vi "TESynC Example.vi"() -> ()   [LabVIEW 2010]
panel:
  in  "VISA resource name":refnum<visa-resource-name>
  out "Alarms":string
  out "Event State Readback(1=ON,0=OFF)":bool
  in  "Event State":bool
  in  "Event number":u8
  out "Actual Humidity Readback (%)":dbl format="%.2f"
  out "Setpoint Humidity Readback(%)":dbl format="%.2f"
  in  "Humidity Setpoint(%)":dbl format="%.2f"
  out "Actual Temp Readback (C)":dbl format="%.2f"
  out "Chamber State Readback(1=ON,0=OFF) 2":bool
  out "Chamber (1=ON,0=OFF)":bool
  in  "Temperature (C":dbl format="%.2f"
  out "Temp Setpoint Readback(C)":dbl format="%.2f"
  out "error out":errorcluster {"code" format="%.0x"}
  in  "error in (no error)":errorcluster
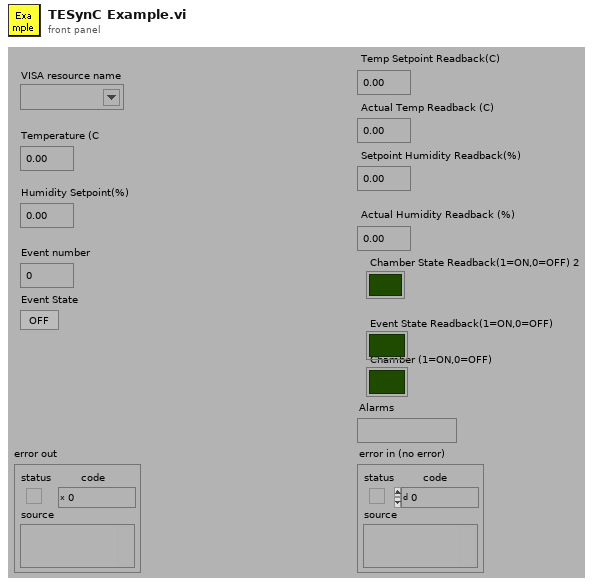
[diagram p1: front panel]
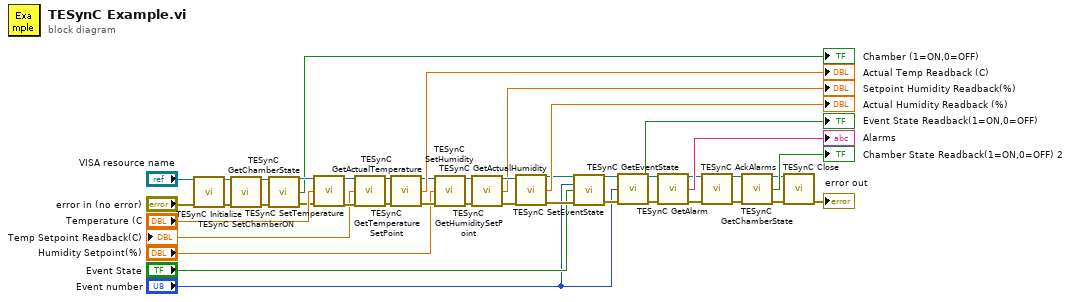
[diagram p0: block diagram]
diagram:
  n1 = call "TESynC Initialize.vi"("VISA resource name"="VISA resource name", "error in (no error)"="error in (no error)") -> ("VISA session"=w37:refnum<visa-resource-name>, "error out"=w38:errorcluster)  [unwired: 12 in]
  n2 = call "TESynC SetChamberON.vi"("VISA session in"=w37, "error in (no error)"=w38) -> ("VISA session out"=w35:refnum<visa-resource-name>, "error out"=w36:errorcluster)  [unwired: 12 in]
  n3 = call "TESynC GetChamberState.vi"("VISA session in"=w35, "error in (no error)"=w36) -> ("VISA session out"=w34:refnum<visa-resource-name>, "Chamber State Readback (1=ON,0=OFF)"=→"Chamber (1=ON,0=OFF)":bool, "error out"=w33:errorcluster)  [unwired: 11 in]
  n4 = call "TESynC SetTemperature.vi"("VISA session in"=w34, "Temperature (C"="Temperature (C", "error in (no error)"=w33) -> ("VISA session out"=w41:refnum<visa-resource-name>, "error out"=w42:errorcluster)  [unwired: 11 in]
  n5 = call "TESynC GetTemperatureSetPoint.vi"("VISA session in"=w41, "error in (no error)"=w42) -> ("VISA session out"=w28:refnum<visa-resource-name>, "Temp Setpoint Readback (C)"=→"Temp Setpoint Readback(C)":dbl, "error out"=w29:errorcluster)  [unwired: 11 in]
  n6 = call "TESynC GetActualTemperature.vi"("VISA session in"=w28, "error in (no error)"=w29) -> ("VISA session out"=w25:refnum<visa-resource-name>, "Actual Temp Readback (C)"=→"Actual Temp Readback (C)":dbl, "error out"=w26:errorcluster)  [unwired: 11 in]
  n7 = call "TESynC SetHumidity.vi"("VISA session in"=w25, "Humidity (%)"="Humidity Setpoint(%)", "error in (no error)"=w26) -> ("VISA session out"=w21:refnum<visa-resource-name>, "error out"=w22:errorcluster)  [unwired: 11 in]
  n8 = call "TESynC GetHumiditySetPoint.vi"("VISA session in"=w21, "error in (no error)"=w22) -> ("VISA session out"=w20:refnum<visa-resource-name>, "Setpoint Humidity Readback(%)"=→"Setpoint Humidity Readback(%)":dbl, "error out"=w23:errorcluster)  [unwired: 11 in]
  n9 = call "TESynC GetActualHumidity.vi"("VISA session in"=w20, "error in (no error)"=w23) -> ("VISA session out"=w16:refnum<visa-resource-name>, "Actual Humidity Readback (%)"=→"Actual Humidity Readback (%)":dbl, "error out"=w17:errorcluster)  [unwired: 11 in]
  n10 = call "TESynC SetEventState.vi"("VISA session in"=w16, "Event number"="Event number", "Event State"="Event State", "error in (no error)"=w17) -> ("VISA session out"=w13:refnum<visa-resource-name>, "error out"=w14:errorcluster)  [unwired: 10 in]
  n11 = call "TESynC GetEventState.vi"("VISA session in"=w13, "Event Number"="Event number", "error in (no error)"=w14) -> ("VISA session out"=w8:refnum<visa-resource-name>, "Event State Readback (1=ON,0=OFF)"=→"Event State Readback(1=ON,0=OFF)":bool, "error out"=w9:errorcluster)  [unwired: 10 in]
  n12 = call "TESynC GetAlarm.vi"("VISA session in"=w8, "error in (no error)"=w9) -> ("VISA session out"=w7:refnum<visa-resource-name>, "Alarms"=→"Alarms":string, "error out"=w6:errorcluster)  [unwired: 11 in]
  n13 = call "TESynC AckAlarms.vi"("VISA session in"=w7, "error in (no error)"=w6) -> ("VISA session out"=w5:refnum<visa-resource-name>, "error out"=w4:errorcluster)  [unwired: 12 in]
  n14 = call "TESynC GetChamberState.vi"("VISA session in"=w5, "error in (no error)"=w4) -> ("VISA session out"=w2:refnum<visa-resource-name>, "Chamber State Readback (1=ON,0=OFF)"=→"Chamber State Readback(1=ON,0=OFF) 2":bool, "error out"=w1:errorcluster)  [unwired: 11 in]
  n15 = call "TESynC Close.vi"("VISA session in"=w2, "error in (no error)"=w1) -> ("error out"=→"error out":errorcluster)  [unwired: 13 in]
